vi "cha constructor.vi"(10 "Channel No.":i32, 11 "Channel Type":T1(ring)) -> (3 "Channel Number":i32)   [LabVIEW 2021, in "libad4.lvlib"]
doc: "Helper to make setting the channel ID easier."
uses:
  <userlib>/libad4/libad4.lvlib
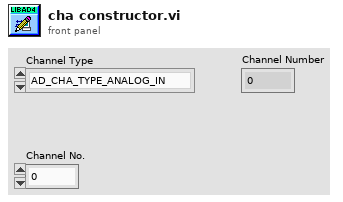
[diagram p1: front panel]
types:
  T1 = enum16{"AD_CHA_TYPE_ANALOG_IN", "AD_CHA_TYPE_ANALOG_OUT", "AD_CHA_TYPE_DIGITAL_IO", "AD_CHA_TYPE_COUNTER"}
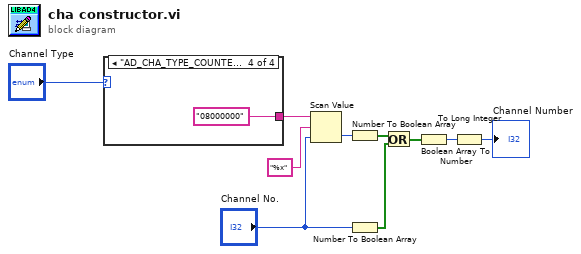
[diagram p0: block diagram]
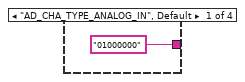
[diagram p2: hidden frame]
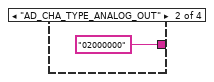
[diagram p3: hidden frame]
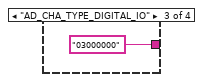
[diagram p4: hidden frame]
diagram:
  n1 = case shown="\"AD_CHA_TYPE_COUNTER\"" "Channel Type" {
    tunnel: ["01000000" "02000000" "03000000" "08000000"] -> w3
    frame "AD_CHA_TYPE_ANALOG_IN", Default {
    }
    frame "AD_CHA_TYPE_ANALOG_OUT" {
    }
    frame "AD_CHA_TYPE_DIGITAL_IO" {
    }
    frame "AD_CHA_TYPE_COUNTER" {
    }
  }
  n2 = Scan Value(string=w3, format string="%x", default (0 dbl)="Channel No.") -> (value=w5:i32)  [unwired: 1 out]
  n3 = Number To Boolean Array(number=w5) -> (Boolean array=w7:bool[])
  n4 = Number To Boolean Array(number="Channel No.") -> (Boolean array=w9:bool[])
  n5 = Or(x=w7, y=w9) -> (x .or. y?=w8:bool[])
  n6 = Boolean Array To Number(Boolean array=w8) -> (number=w2:i32)
  n7 = To Long Integer(number=w2) -> (32bit integer=→"Channel Number":i32)
